vi "Create-unique-queue.vi"(8 "error in (no error)":errorcluster, 10 "Prefix":string) -> (0 "error out":errorcluster, 2 "ID":i32, 3 "Queue out":refnum<queue>)   [LabVIEW 2013, in "SLMServer.lvlib" / "SLMServer.lvclass"]
uses:
  SLMServer.lvclass
  SA-SLMAPI/Sources/Message.lvclass
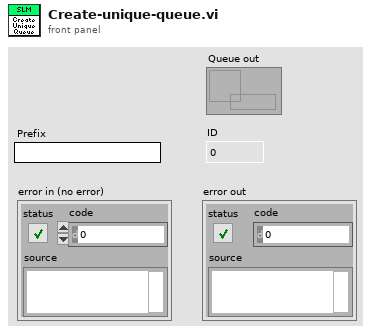
[diagram p1: front panel]
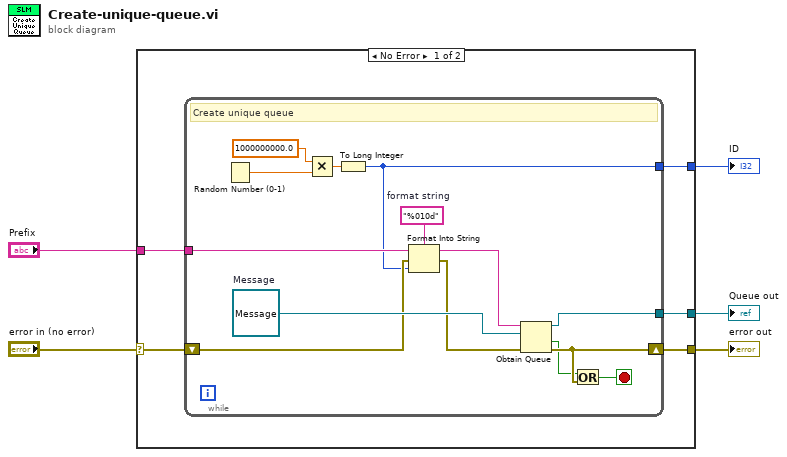
[diagram p0: block diagram]
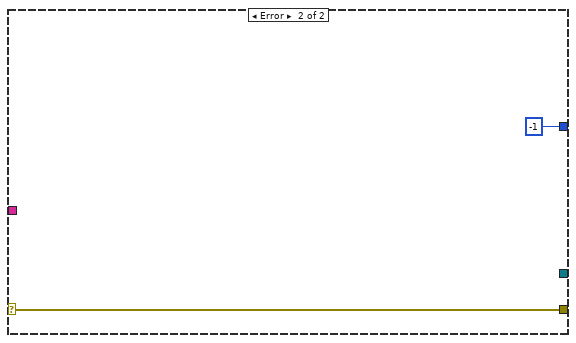
[diagram p2: hidden frame]
diagram:
  n1 = case shown="No Error" "error in (no error)" {
    selector: "error in (no error)" -> [w6 w26]
    tunnel: [w10 -1] -> w5
    tunnel: "Prefix" -> [w9 _]
    tunnel: [w8 _] -> w3
    tunnel: [w7 w26] -> w2
    frame No Error {
      n2 = while {
        shift-right: [w22] -> w7
        shift-left: w6 -> [w16]
        tunnel: [w13] -> w8
        tunnel: w9 -> [w12]
        tunnel: [w11] -> w10
        stop <- w23 stop-if-true
        w18 = "%010d"  # format string
        w24 = refnum<class "Message.lvclass"> refnum  # Message
        # "Create unique queue"
        n3 = Random Number (0-1)() -> (number: 0 to 1=w20:dbl)
        n4 = Multiply(x=1000000000.0, y=w20) -> (x*y=w17:dbl)
        n5 = To Long Integer(number=w17) -> (32bit integer=w11:i32)
        n6 = Format Into String(format string=w18, initial string=w12, error in=w16, w11) -> (resulting string=w14:string, error out=w15:errorcluster)
        n7 = Obtain Queue(name (unnamed)=w14, element data type=w24, error in (no error)=w15) -> (queue out=w13:refnum<queue>, created new?=w21:bool, error out=w22:errorcluster)  [unwired: 2 in]
        n8 = Or(x=w21, y=w22) -> (x .or. y?=w23:bool)
      }
    }
    frame Error {
    }
  }
  "ID" <- w5
  "Queue out" <- w3
  "error out" <- w2
